vi "Tx Ch FIFO Count.vi"(9 "FIFOCount":u32, 10 "Channel":u8, 11 "devId":i32) -> (1 "FIFOCount out":u32, 2 "devId out":i32, 3 "function return":i32)   [LabVIEW 2013, in "CHR34XXX.lvlib"]
doc: "DLL BOOL __stdcall CHR34XXX_TxCh_SetMode(IN int devId,IN BYTE Channel,IN BYTE Mode); DLL BOOL __stdcall CHR34XXX_TxCh_SetPeriod(IN int devId,IN BYTE Channel,IN DWORD Period); DLL BOOL __stdcall CHR34XXX_TxCh_FIFOState(IN int devId,IN BYTE Channel,OUT DWORD *State); DLL BOOL __stdcall CHR34XXX_TxCh_FIFOCount(IN int devId,IN BYTE Channel,OUT DWORD *FIFOCount);"
uses:
  CHR34XXX.lvlib
  CHR34XXX.dll
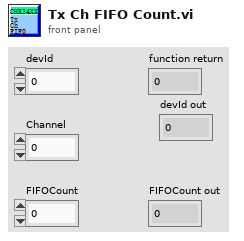
[diagram p1: front panel]
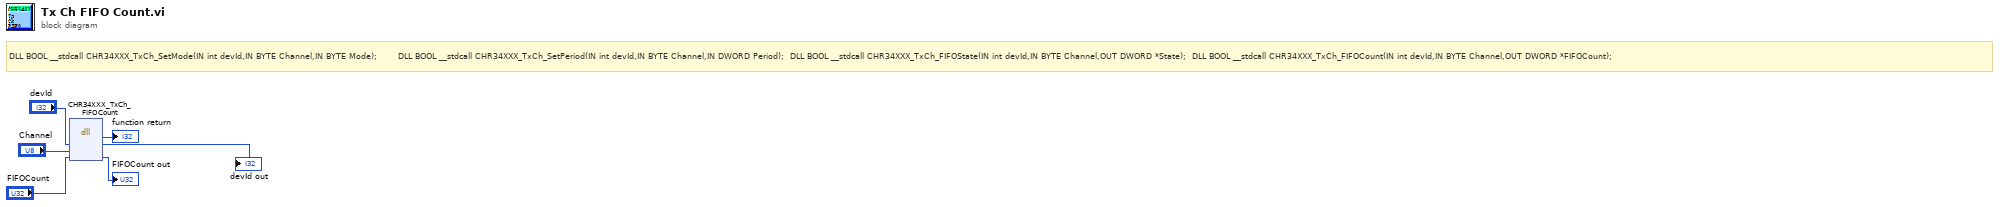
[diagram p0: block diagram]
diagram:
  # "DLL BOOL __stdcall CHR34XXX_TxCh_SetMode(IN int devId,IN BYTE Channel,IN BYTE Mode);       DLL BOOL __stdcall CHR34XXX_TxCh_SetPeriod(IN int devId,IN BYTE Channel,IN DWORD Period);  DLL BOOL __stdcall CHR34XXX_TxCh_FIFOState(IN int devId,IN BYTE Channel,OUT DWORD *State);  DLL BOOL __stdcall CHR34XXX_TxCh_FIFOCount(IN int devId,IN BYTE Channel,OUT DWORD *FIFOCount);"
  n1 = dll-call lib="C:/Users/dy/Desktop/CHR34XXX_lv/lv_lib/CHR34XXX.*" fn="CHR34XXX_TxCh_FIFOCount"("devId"="devId", "Channel"="Channel", "FIFOCount"="FIFOCount") -> (→"function return":i32, "devId"=→"devId out":i32, "FIFOCount"=→"FIFOCount out":u32)  [unwired: 4 in, 2 out]
